vi "DequeueElement.vi"(8 "error in (no error)":errorcluster, 11 "QueueIN":refnum<queue>) -> (0 "error out":errorcluster, 1 "Data":variant, 2 "Actions":string, 3 "QueueOUT":refnum<queue>)   [LabVIEW 2018]
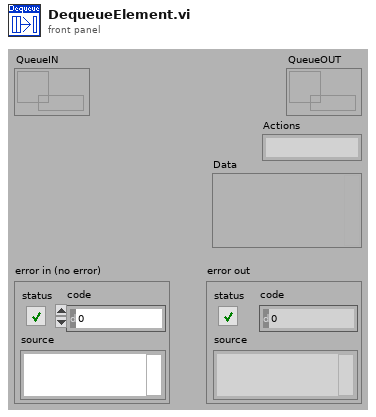
[diagram p1: front panel]
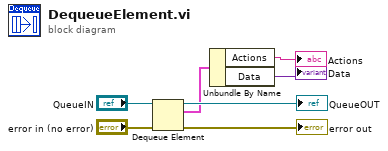
[diagram p0: block diagram]
diagram:
  n1 = Dequeue Element(queue="QueueIN", error in (no error)="error in (no error)") -> (queue out=→"QueueOUT":refnum<queue>, element=w5:cluster{"Actions":string, "Data":variant}, error out=→"error out":errorcluster)  [unwired: 2 out]
  n2 = Unbundle By Name(w5) -> ("Actions"=→"Actions":string, "Data"=→"Data":variant)
